vi "Connect.vi"(8 "error in":errorcluster, 11 "DIG_IO in":refnum<class "DIG_IO.lvclass">) -> (0 "error out":errorcluster, 3 "DIG_IO out":refnum<class "DIG_IO.lvclass">)   [LabVIEW 2019, in "DIG_IO.lvlib" / "DIG_IO.lvclass"]
doc: "This override VI is a carryover override from the parent class, children classes *must* override this VI and therefore the parent class must contain this VI to maintain the override rules."
uses:
  Library/DIG_IO.lvclass
  builds/Instruments/Instruments.lvlibp/Library/Instruments.lvclass
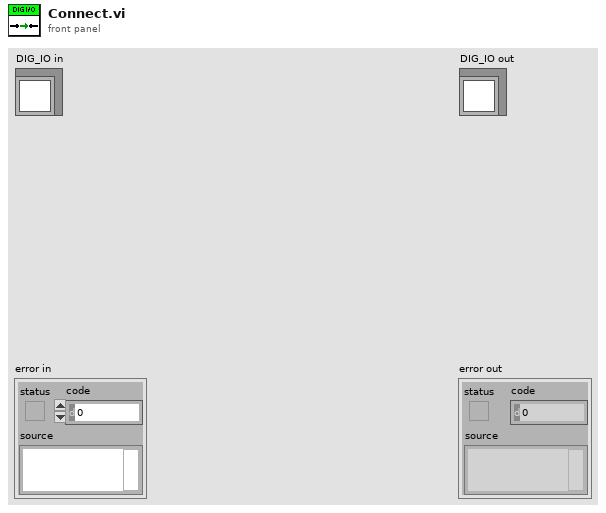
[diagram p1: front panel]
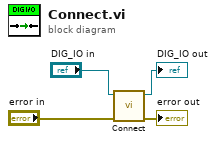
[diagram p0: block diagram]
diagram:
  n1 = call-parent "Connect.vi"("error in (no error)"="error in", "Instruments in"="DIG_IO in") -> ("error out"=→"error out":errorcluster, "Instruments out"=→"DIG_IO out":refnum<class "DIG_IO.lvclass">)  [unwired: 8 in]
